vi "Generate top-level name prefixes.vi"(8 "error in":errorcluster, 9 "Add Prefix?":bool=TRUE, 10 "Container - Regex pairs":T1=[{"Container to create"="TEST", "Regex"="^test_.*\\.vi"}, {"Container to create"="TEST", "Regex"="_test.vi$"}, {"Container to create"="DRV", "Regex"="^DRV_.*\\.lv.*$"}, {"Container to create"="HWT", "Regex"="^HWT_.*\\.lv.*$"}, {"Container to create"="FCN", "Regex"="^FCN_.*\\.lv.*$"}, {"Container to create"="INS", "Regex"="^INS_.*\\.lv.*$"}], 11 "String":string) -> (0 "error out":errorcluster, 3 "element":string)   [LabVIEW 2018, in "Shared Dependencies.lvlib"]
uses:
  Shared Dependencies/Shared Dependencies.lvlib
  Shared Dependencies/Container - Regex array.ctl
  Dep Names and Paths.ctl
  Name and Dependency Processing.lvlib
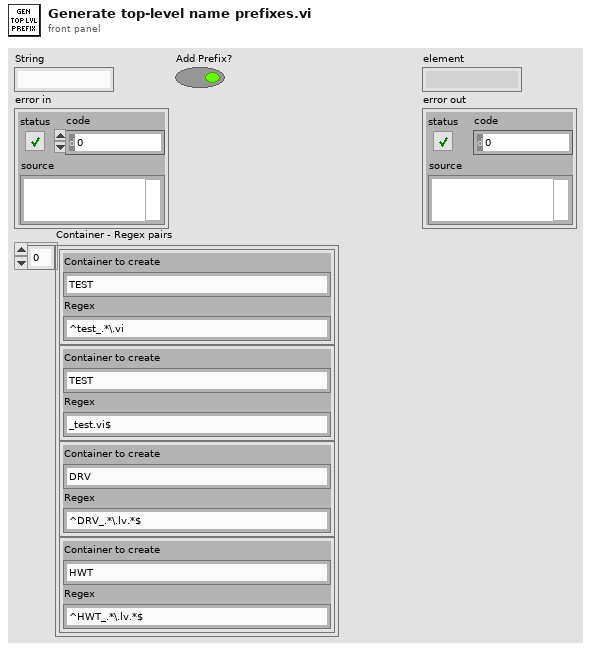
[diagram p1: front panel]
types:
  T1 = typedef "Shared Dependencies.lvlib/Container - Regex array.ctl" = cluster{"Container to create":string, "Regex":string}[]
  T2 = typedef "Name and Dependency Processing.lvlib/Dep Names and Paths.ctl" = cluster{"Dependency Names":string[], "Dependency Paths":path[]}
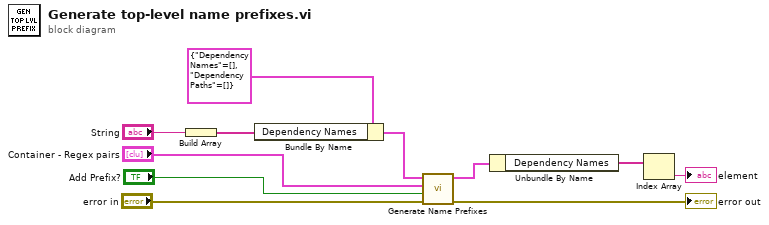
[diagram p0: block diagram]
diagram:
  n1 = Build Array("String") -> (w10:string[])
  n2 = Bundle By Name(cluster=T2 {"Dependency Names"=[], "Dependency Paths"=[]} ("Dep Names and Paths"), "Dependency Names"=w10) -> (w8:T2)
  n3 = call "Generate Name Prefixes.vi"("error in"="error in", "Add Prefix?"="Add Prefix?", "Container - Regex pairs"="Container - Regex pairs", "Dep Names and Paths"=w8) -> ("error out"=→"error out":errorcluster, "Prefixed Dep Names and Paths"=w7:T2)  [unwired: 6 in]
  n4 = Unbundle By Name(w7) -> ("Dependency Names"=w6:string[])
  n5 = Index Array(array=w6) -> (element=→"element":string)  [unwired: 1 in]
